vi "Hex2Signed.vi"(1 "IN":dbl) -> (0 "OUT":dbl)   [LabVIEW 2024]
doc: "Conversión de Hexadecimal a Entero"
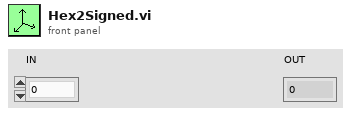
[diagram p1: front panel]
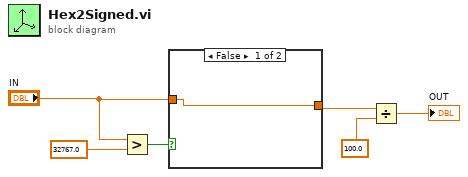
[diagram p0: block diagram]
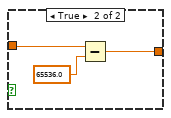
[diagram p2: hidden frame]
diagram:
  n1 = Greater?(x="IN", y=32767.0) -> (0:w5:bool)
  n2 = case shown="False" w5 {
    tunnel: "IN" -> [w7 w10]
    tunnel: [w7 w8] -> w3
    frame False {
    }
    frame True {
      n3 = Subtract(x=w10, y=65536.0) -> (x-y=w8:dbl)
    }
  }
  n4 = Divide(x=w3, y=100.0) -> (x/y=→"OUT":dbl)
